vi "To Origin File dYdX.vi"(4 "Y":dbl[](array[numeric]), 6 "dYdX":dbl[](array[numeric]), 8 "X":dbl[](array[numeric]), 10 "Postfix":string, 11 "Prefix":string) -> (3 "Text":string)   [LabVIEW 2018]
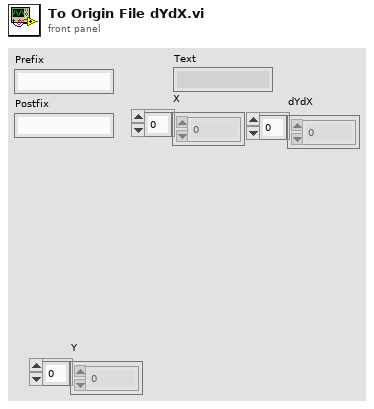
[diagram p1: front panel]
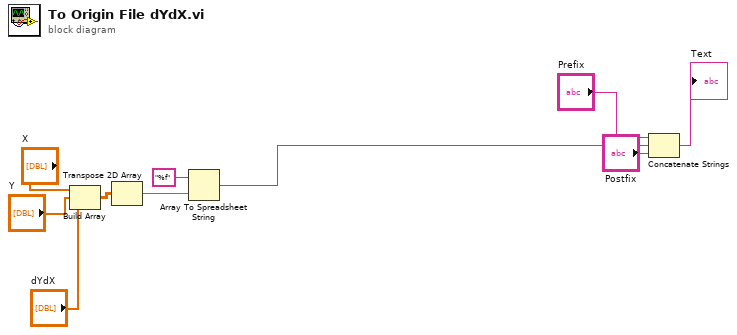
[diagram p0: block diagram]
diagram:
  n1 = Build Array("X", "Y", "dYdX") -> (w8:dbl[][])
  n2 = Transpose 2D Array(2D array=w8) -> (transposed array=w9:dbl[][])
  n3 = Array To Spreadsheet String(array=w9, 3:"%f" ("format string")) -> (spreadsheet string=w3:string)  [unwired: 1 in]
  n4 = Concatenate Strings("Prefix", w3, "Postfix") -> (→"Text":string)
